vi "Configure TCP Server Connection.vi"(5 "Connection.TCP":refnum<class "Connection.TCP.lvclass">, 6 "timeout (5000ms)":i32=5000, 8 "error in (no error)":errorcluster, 10 "remote port (80)":u16=80) -> (0 "error out":errorcluster, 3 "Connection.TCP":refnum<class "Connection.TCP.lvclass">)   [LabVIEW 2013, in "Connection.TCP_GOSPL.lvlib" / "Connection.TCP.lvclass"]
uses:
  Connection.TCP.lvclass
  Connection/Connection.lvclass/Connection.ctl
  Connection/Connection.lvclass
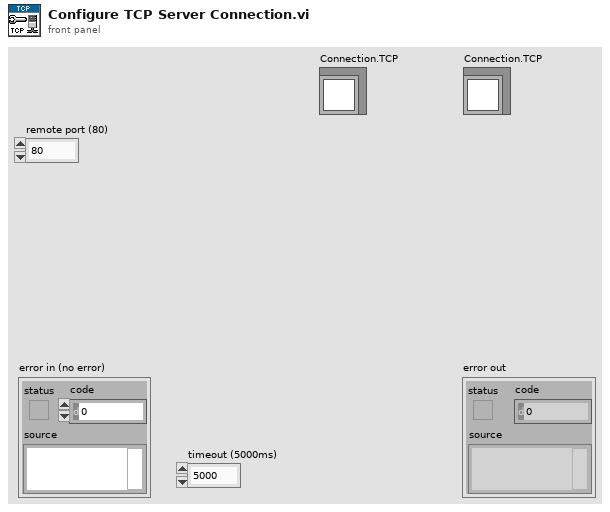
[diagram p1: front panel]
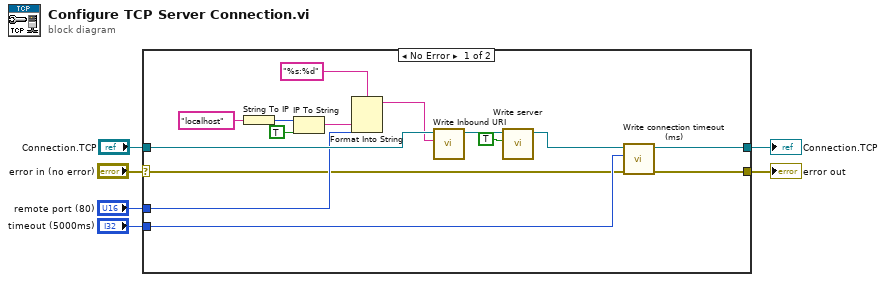
[diagram p0: block diagram]
diagram:
  n1 = case shown="No Error" "error in (no error)" {
    selector: "error in (no error)" -> [w11 w23]
    tunnel: [w19 w23] -> w5
    tunnel: [w20 w22] -> w2
    tunnel: "remote port (80)" -> [w15 _]
    tunnel: "timeout (5000ms)" -> [w21 _]
    tunnel: "Connection.TCP" -> [w17 w22]
    frame No Error {
      n2 = String To IP(1:"localhost" ("name")) -> (0:w10:u32)
      n3 = IP To String(1:TRUE ("dot notation? (F)"), 2:w10) -> (0:w8:string)
      n4 = Format Into String(format string="%s:%d" ("Inbound URI"), w8, w15) -> (resulting string=w13:string)  [unwired: 2 in, 1 out]
      n5 = call "Write Inbound URI.vi"("Inbound URI"=w13, "Connection in"=w17) -> ("Connection out"=w16:refnum<class "Connection.TCP.lvclass">)  [unwired: 9 in]
      n6 = call "Write server.vi"("server"=TRUE, "Connection in"=w16) -> ("Connection out"=w12:refnum<class "Connection.TCP.lvclass">)  [unwired: 9 in]
      n7 = call "Write connection timeout (ms).vi"("error in (no error)"=w11, "connection timeout (ms)"=w21, "Connection in"=w12) -> ("error out"=w19:errorcluster, "Connection out"=w20:refnum<class "Connection.TCP.lvclass">)  [unwired: 7 in]
    }
    frame Error {
    }
  }
  "error out" <- w5
  "Connection.TCP" <- w2
